vi "Ejercicio_16_histeresis.vi"() -> ()   [LabVIEW 2020]
panel:
  in  "stop":bool
  out "Boolean":bool
  in  "Sensor":dbl
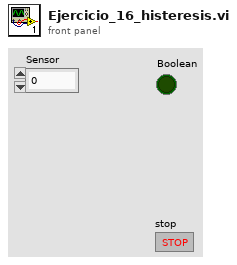
[diagram p1: front panel]
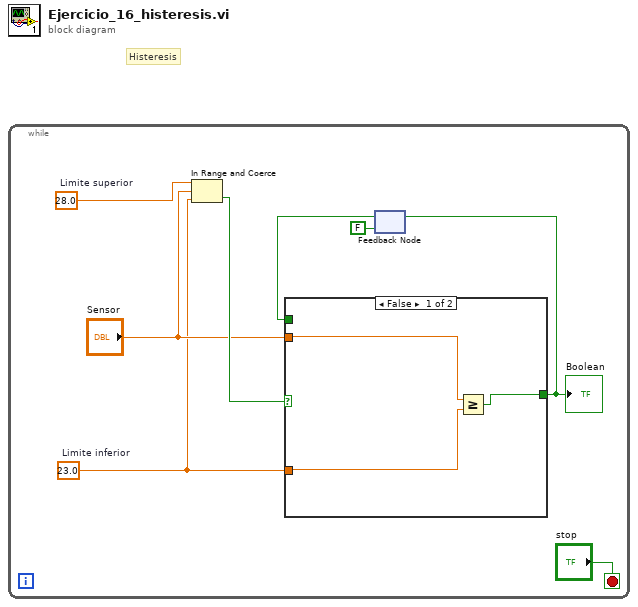
[diagram p0: block diagram]
diagram:
  # "Histeresis"
  n1 = while {
    stop <- "stop" stop-if-true
    w1 = 23.0  # Limite inferior
    w8 = 28.0  # Limite superior
    n2 = In Range and Coerce(upper limit=w8, x="Sensor", lower limit=w1) -> (In Range?=w6:bool)  [unwired: 1 out]
    n3 = feedback #1(FALSE) -> (w7:bool)
    n4 = case shown="False" w6 {
      tunnel: "Sensor" -> [w11 _]
      tunnel: w1 -> [w10 _]
      tunnel: w7 -> [_ w12]
      tunnel: [w9 w12] -> w4
      frame False {
        n5 = Greater Or Equal?(x=w11, y=w10) -> (x >= y?=w9:bool)
      }
      frame True {
      }
    }
    "Boolean" <- w4
    n6 = feedback-in #1(w4) -> ()
  }
